vi "rus fit - filter all.vi"(6 "filter window (kHz)":dbl=40.0 caption="(kHz)", 10 "omega":dbl[](array[numeric]), 11 "Array":cdb[](array[numeric])) -> (3 "Array out":cdb[](array[numeric]))   [LabVIEW 2010]
uses:
  <vilib>/Analysis/3filter.llb/Filter Passband Type.ctl
  <vilib>/Analysis/NI_AALBase.lvlib
  <vilib>/Analysis/3filter.llb/FIR Windowed Filter (DBL).vi
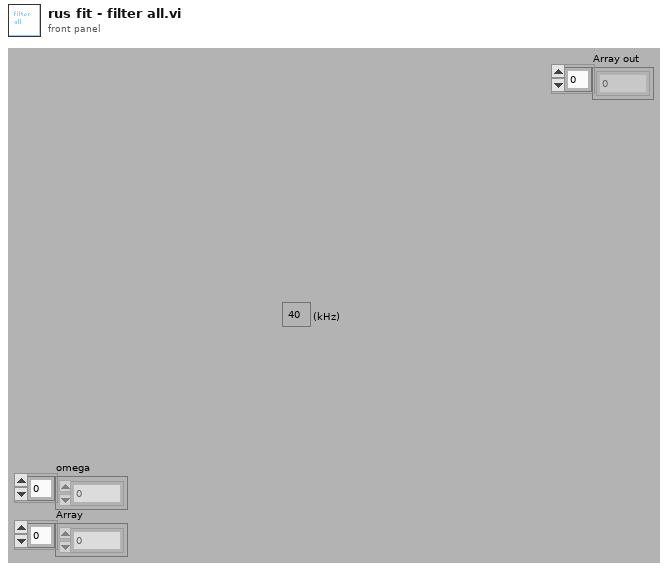
[diagram p1: front panel]
types:
  T1 = typedef "NI_AALBase.lvlib/Filter Passband Type.ctl" = enum32{"Lowpass", "Highpass", "Bandpass", "Bandstop"}
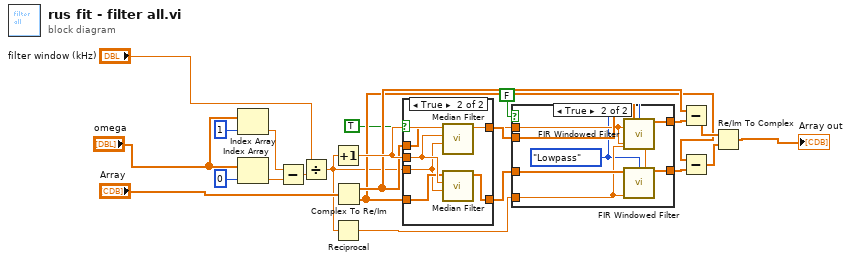
[diagram p0: block diagram]
diagram:
  n1 = Index Array(array="omega", index=1) -> (element=w14:dbl)
  n2 = Index Array(array="omega", index=0) -> (element=w13:dbl)
  n3 = Subtract(x=w14, y=w13) -> (x-y=w12:dbl)
  n4 = Divide(x="filter window (kHz)", y=w12) -> (x/y=w3:dbl)
  n5 = Increment(x=w3) -> (x+1=w6:dbl)
  n6 = Reciprocal(x=w3) -> (1/x=w7:dbl)
  n7 = Complex To Re/Im(x + iy="Array") -> (x=w5:dbl[], y=w4:dbl[])
  n8 = case shown="True" TRUE {
    tunnel: [w24 w30] -> w11
    tunnel: [w23 w29] -> w9
    tunnel: w6 -> [_ w28]
    tunnel: w5 -> [w24 w27]
    tunnel: w4 -> [w23 w26]
    tunnel: w3 -> [_ w25]
    frame False {
    }
    frame True {
      n9 = call <vilib>:"Median Filter.vi"("right rank"=w25, "left rank"=w28, "X"=w27) -> ("Filtered X"=w30:dbl[])  [unwired: 7 in, 1 out]
      n10 = call <vilib>:"Median Filter.vi"("right rank"=w25, "left rank"=w28, "X"=w26) -> ("Filtered X"=w29:dbl[])  [unwired: 7 in, 1 out]
    }
  }
  n11 = case shown="True" FALSE {
    tunnel: w11 -> [w32 w39]
    tunnel: [w32 w38] -> w10
    tunnel: w9 -> [w31 w37]
    tunnel: [w31 w36] -> w8
    tunnel: w7 -> [_ w35]
    tunnel: w6 -> [_ w34]
    frame False {
    }
    frame True {
      w33 = Filter_Passband_Type."Lowpass" ("filter type")
      n12 = call-poly <vilib>:"FIR Windowed Filter.vi"("X"=w39, "filter type"=w33, "window parameter"=w34, "high cutoff freq: fh"=w35) -> ("Filtered X"=w38:dbl[])  [unwired: 10 in, 1 out]
      n13 = call-poly <vilib>:"FIR Windowed Filter.vi"("X"=w37, "filter type"=w33, "window parameter"=w34, "high cutoff freq: fh"=w35) -> ("Filtered X"=w36:dbl[])  [unwired: 10 in, 1 out]
    }
  }
  n14 = Subtract(x=w5, y=w10) -> (x-y=w18:dbl[])
  n15 = Subtract(x=w4, y=w8) -> (x-y=w17:dbl[])
  n16 = Re/Im To Complex(1:w17, 2:w18) -> (0:→"Array out":cdb[])
